vi "checkTime.vi"(8 "error (in)":errorcluster, 11 "Data (in)":T7) -> (0 "error (out)":errorcluster, 2 "Required Delay":dbl, 3 "Data (out)":T7)   [LabVIEW 2015]
doc: "Check time to ensure that a delay can be made if necessary to prevent the actuator from overheating."
uses:
  <vilib>/MakerHub/LINX/Private/Type Defs/LINX Ref.ctl
  <vilib>/MakerHub/LINX/Private/Type Defs/Platform.ctl
  <vilib>/MakerHub/LINX/Private/Type Defs/Interface.ctl
  <vilib>/MakerHub/LINX/Private/Device/Type Defs/LINX Device Config.ctl
  <vilib>/MakerHub/LINX/Private/Device/Type Defs/TCP Config.ctl
  <vilib>/MakerHub/LINX/Private/Device/Type Defs/Channels.ctl
  <vilib>/MakerHub/LINX/LMH-LINX.lvlib
  <vilib>/MakerHub/LINX/Private/Device/Device.lvlib
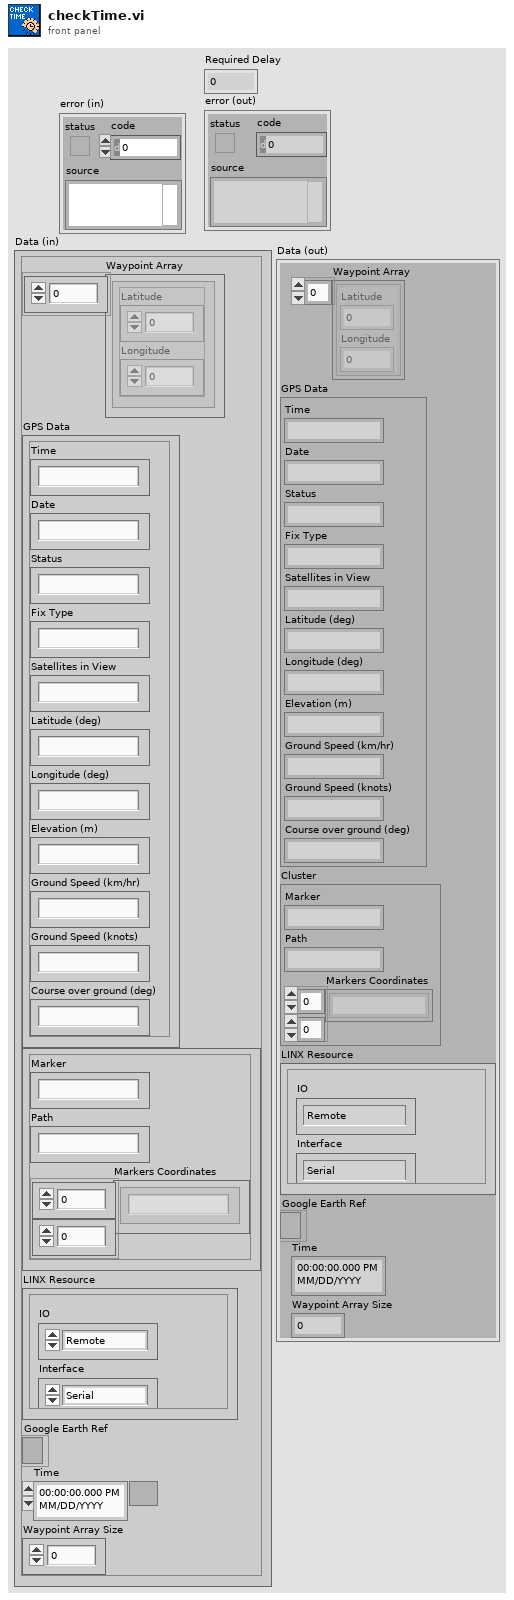
[diagram p1: front panel]
types:
  T1 = typedef "LMH-LINX.lvlib/LINX Ref.ctl" = cluster{"IO":T2, "Interface":T3, "LINX Device Config":T4}
  T2 = typedef "LMH-LINX.lvlib/Platform.ctl" = enum16{"Remote", "Local"}
  T3 = typedef "LMH-LINX.lvlib/Interface.ctl" = enum16{"Serial", "TCP"}
  T4 = typedef "LMH-LINX.lvlib/Device.lvlib/LINX Device Config.ctl" = cluster{"Interface":T3, "COM Port":refnum<visa-resource-name>, "TCP Configuration":T5, "Device Family":u8, "Device ID":u8, "Device Name":string, "TCP Ref":refnum<k5>, "Channels":T6}
  T5 = typedef "LMH-LINX.lvlib/Device.lvlib/TCP Config.ctl" = cluster{"IP Address":string, "Port":u16}
  T6 = typedef "LMH-LINX.lvlib/Channels.ctl" = cluster{"DI":u8[], "DO":u8[], "AI":u8[], "AO":u8[], "PWM":u8[], "QE":u8[], "UART":u8[], "I2C 2":u8[], "SPI":u8[], "CAN":u8[], "Servo":u8[], "AI Ref (V)":dbl, "AI Resolution (Bits)":u8, "AO Ref (V)":dbl, "AO Resolution (Bits)":u8}
  T7 = cluster{"Waypoint Array":cluster{"Latitude":dbl, "Longitude":dbl}[], "GPS Data":cluster{"Time":string, "Date":string, "Status":string, "Fix Type":string, "Satellites in View":string, "Latitude (deg)":string, "Longitude (deg)":string, "Elevation (m)":string, "Ground Speed (km/hr)":string, "Ground Speed (knots)":string, "Course over ground (deg)":string}, "Cluster":cluster{"Marker":string, "Path":string, "Markers Coordinates":string[][]}, "LINX Resource":T1, "Google Earth Ref":refnum<k7>, "Time":timestamp, "Waypoint Array Size":i32}
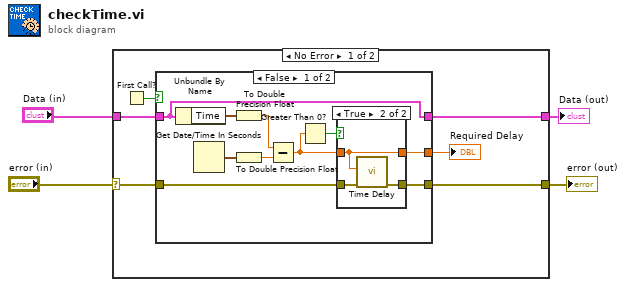
[diagram p0: block diagram]
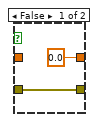
[diagram p2: hidden frame]
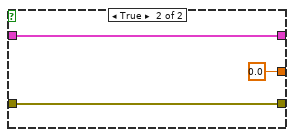
[diagram p3: hidden frame]
diagram:
  n1 = case shown="No Error" "error (in)" {
    selector: "error (in)" -> [w6 w30]
    tunnel: [w5 w30] -> w4
    tunnel: "Data (in)" -> [w10 w29]
    tunnel: [w8 w29] -> w1
    frame No Error {
      n2 = First Call?() -> (First Call?: T/F=w9:bool)
      n3 = case shown="False" w9 {
        tunnel: w10 -> [w18 w28]
        tunnel: [w18 w28] -> w8
        tunnel: [w13 0.0] -> w7
        tunnel: w6 -> [w12 w26]
        tunnel: [w11 w26] -> w5
        frame False {
          n4 = Unbundle By Name(w18) -> ("Time"=w20:timestamp)
          n5 = Get Date/Time In Seconds() -> (seconds since 1Jan1904=w19:timestamp)
          n6 = To Double Precision Float(number=w20) -> (double precision float=w17:dbl)
          n7 = To Double Precision Float(number=w19) -> (double precision float=w16:dbl)
          n8 = Subtract(x=w17, y=w16) -> (x-y=w14:dbl)
          n9 = Greater Than 0?(x=w14) -> (x > 0?=w15:bool)
          n10 = case shown="True" w15 {
            tunnel: w14 -> [_ w23]
            tunnel: [0.0 w23] -> w13
            tunnel: w12 -> [w22 w25]
            tunnel: [w22 w24] -> w11
            frame False {
            }
            frame True {
              n11 = call "Time Delay"("error in (no error)"=w25, "Delay Time (s)"=w23) -> ("error out"=w24:errorcluster)  [unwired: 9 in]
            }
          }
        }
        frame True {
        }
      }
      "Required Delay" <- w7
    }
    frame Error {
    }
  }
  "error (out)" <- w4
  "Data (out)" <- w1
